vi "Vollbremsloop.vi"(11 "Queue in":refnum<queue>) -> ()   [LabVIEW 2016]
uses:
  Globale Variablen VI/AutonomousMode.vi
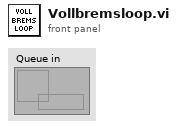
[diagram p1: front panel]
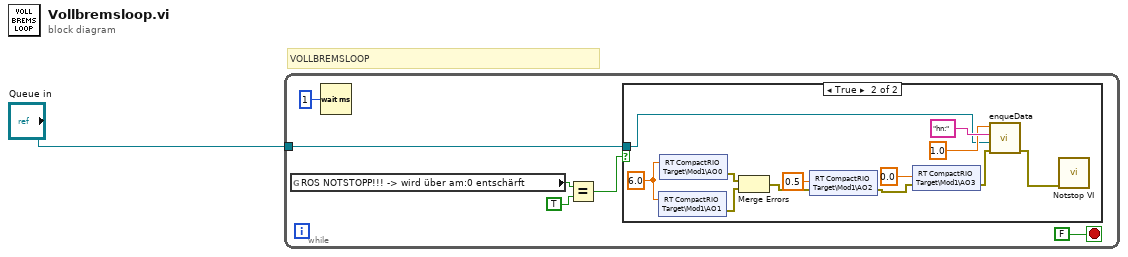
[diagram p0: block diagram]
diagram:
  # "VOLLBREMSLOOP"
  n1 = while {
    tunnel: "Queue in" -> [w4]
    stop <- FALSE stop-if-true
    n2 = global read "AutonomousMode.vi" "ROS NOTSTOPP!!! -> wird über am:0 entschärft"() -> (w5:bool)
    n3 = Wait (ms)(milliseconds to wait=u32 1) -> ()  [unwired: 1 out]
    n4 = Equal?(x=w5, y=TRUE) -> (x = y?=w3:bool)
    n5 = case shown="True" w3 {
      tunnel: w4 -> [_ w8]
      frame False {
      }
      frame True {
        w17 = 6.0
        n6 = shared-variable "RT CompactRIO Target\\Mod1\\AO1"(w17) -> (error out=w16:errorcluster)  [unwired: 1 in]
        n7 = shared-variable "RT CompactRIO Target\\Mod1\\AO0"(w17) -> (error out=w15:errorcluster)  [unwired: 1 in]
        n8 = Merge Errors(w15, w16) -> (w14:errorcluster)
        n9 = shared-variable "RT CompactRIO Target\\Mod1\\AO2"(0.5, error in=w14) -> (error out=w11:errorcluster)
        n10 = shared-variable "RT CompactRIO Target\\Mod1\\AO3"(0.0, error in=w11) -> (error out=w10:errorcluster)
        n11 = call "enqueData.vi"("error in (no error)"=w10, "Queue Reference"=w8, "Descriptor"="hn:", "Value IN"=1.0) -> ("error out"=w9:errorcluster)  [unwired: 7 in]
        n12 = call "Notstop VI.vi"("error in"=w9) -> ()  [unwired: 10 in, 1 out]
      }
    }
  }
